vi "Initialize - Device Sections and Channels.vi"(8 "error in (no error)":errorcluster, 11 "Item Ref out":T1 format="%.0x") -> (0 "error out":errorcluster, 3 "Parent Ref out":T1 format="%.0x")   [LabVIEW 2016, in "UDP-Custom-Device System Explorer.lvlib"]
doc: "Add Status Channels and Receive (Rx) Channels Section to the system definition."
uses:
  UDP-Custom-Device System Explorer.lvlib
  <vilib>/NI Veristand/Custom Device API/Custom Device Item Ref.ctl
  Shared/Constants.vi
  <vilib>/NI VeriStand/Custom Device API/Custom Device API.lvlib
  Shared/UDP-Custom-Device Shared.lvlib
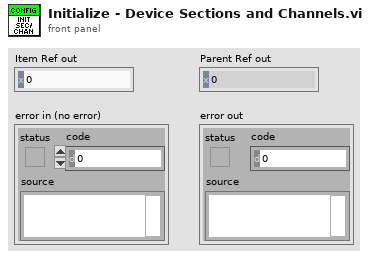
[diagram p1: front panel]
types:
  T1 = typedef "Custom Device API.lvlib/Custom Device Item Ref.ctl" = u64
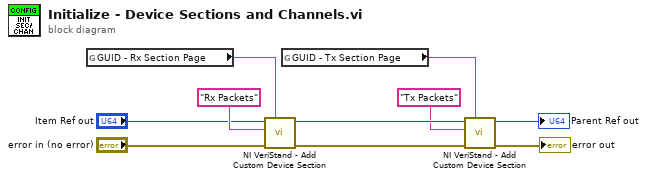
[diagram p0: block diagram]
diagram:
  n1 = global read "Constants.vi" "GUID - Rx Section Page"() -> (w6:string)
  n2 = call <vilib>:"NI VeriStand - Add Custom Device Section.vi"("GUID (Default Section)"=w6, "error in (no error)"="error in (no error)", "Section Name"="Rx Packets", "Parent Ref in"="Item Ref out") -> ("error out"=w8:errorcluster, "Parent Ref out"=w9:T1)  [unwired: 4 in, 2 out]
  n3 = global read "Constants.vi" "GUID - Tx Section Page"() -> (w5:string)
  n4 = call <vilib>:"NI VeriStand - Add Custom Device Section.vi"("GUID (Default Section)"=w5, "error in (no error)"=w8, "Section Name"="Tx Packets", "Parent Ref in"=w9) -> ("error out"=→"error out":errorcluster, "Parent Ref out"=→"Parent Ref out":T1)  [unwired: 4 in, 2 out]
